vi "Orifice Flow Calculator of Water In Evaporation ASME.vi"(2 "Pipe Diameter (mm)":dbl[unit], 3 "Orifice Diameter":dbl[unit], 4 "Delta P\n(Presure Made By Orifice)":dbl[unit], 5 "Water Temperature":dbl[unit]=10.0 min=10.0 max=95.0) -> (0 "Iteration Volumetric Flow \n(Orifice) (Lit/min)":dbl[unit], 1 "Mass Flow (Orifice) (Kg/min)":dbl[unit])   [LabVIEW 2018]
panel:
  out "ReD":dbl
  out "Mass Flow (Orifice) (Kg/h)":dbl[unit](knob)
  out "Mass Flow (Orifice) (Kg/s)":dbl[unit]
  out "Pipe Velocity (m/s)":dbl[unit]
  out "Pipe Area (cm^2)":dbl[unit]
  out "Throat Velocity (m/s)":dbl[unit]
  out "Throat Area (cm^2)":dbl[unit]
  out "Beta":dbl
  out "orifice coefficient":dbl
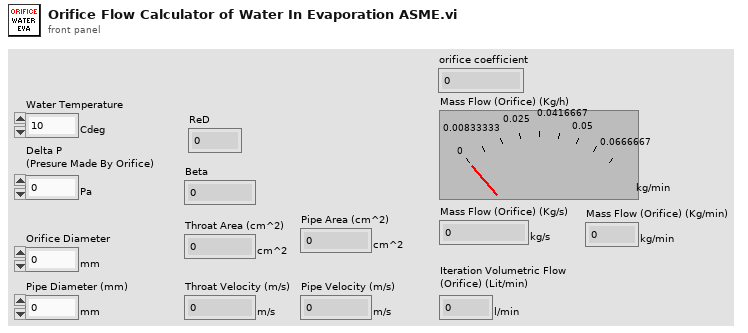
[diagram p1: front panel]
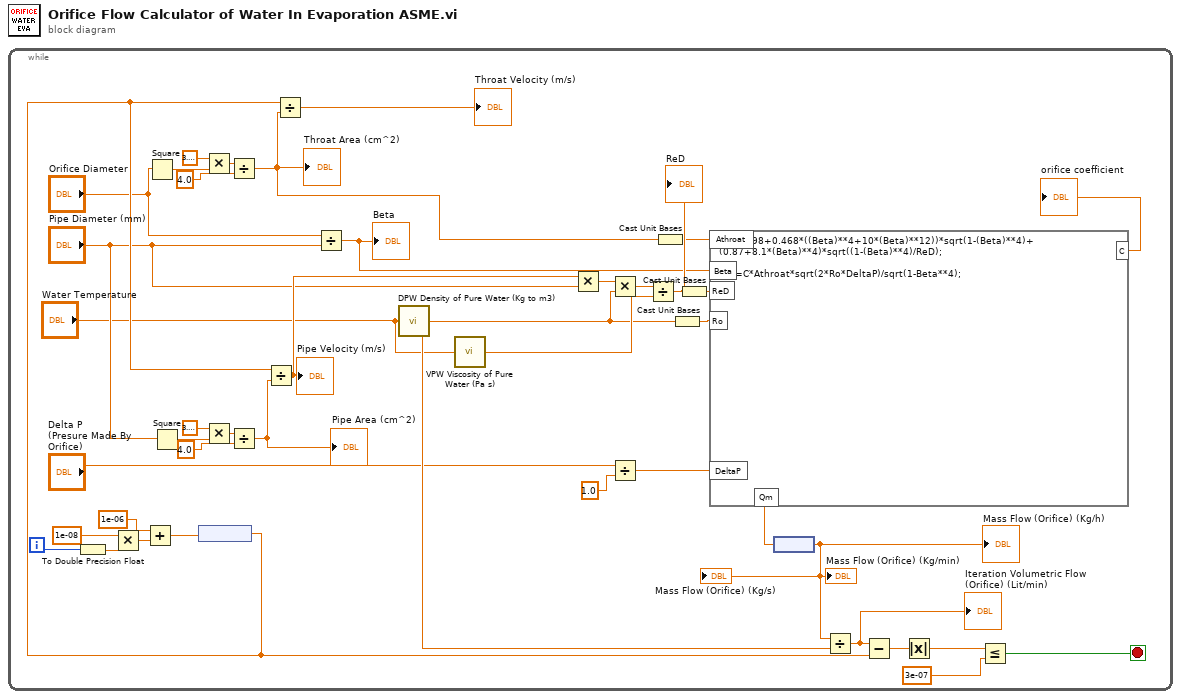
[diagram p0: block diagram]
diagram:
  n1 = while {
    i -> [w26]
    stop <- w19 stop-if-true
    n2 = To Double Precision Float(number=w26) -> (double precision float=w30:dbl)
    n3 = Multiply(x=1e-08, y=w30) -> (x*y=w28:dbl)
    n4 = Add(x=1e-06, y=w28) -> (x+y=w24:dbl)
    n5 = Square(x="Orifice Diameter") -> (x^2=w39:dbl[unit])
    n6 = Square(x="Pipe Diameter (mm)") -> (x^2=w35:dbl[unit])
    n7 = node(w24) -> (w23:dbl[unit])
    n8 = Multiply(x=3.141592653589793, y=w39) -> (x*y=w41:dbl[unit])
    n9 = Multiply(x=3.141592653589793, y=w35) -> (x*y=w37:dbl[unit])
    n10 = Divide(x=w41, y=4.0) -> (x/y=w11:dbl[unit])
    "Throat Area (cm^2)" <- w11
    n11 = Divide(x=w37, y=4.0) -> (x/y=w34:dbl[unit])
    "Pipe Area (cm^2)" <- w34
    n12 = Divide(x=w23, y=w34) -> (x/y=w7:dbl[unit])
    "Pipe Velocity (m/s)" <- w7
    n13 = Divide(x=w23, y=w11) -> (x/y=→"Throat Velocity (m/s)":dbl[unit])
    n14 = Divide(x="Orifice Diameter", y="Pipe Diameter (mm)") -> (x/y=w1:dbl)
    "Beta" <- w1
    n15 = call "DPW Density of Pure Water (Kg to m3).vi"("Pure Water Temprature"="Water Temperature") -> ("DPW"=w8:dbl[unit])
    n16 = call "VPW Viscosity of Pure Water (Pa s).vi"("Pure Water Temprature"="Water Temperature") -> ("Visocity of pure Water (Pa S)"=w13:dbl[unit])
    n17 = Multiply(x=w7, y="Pipe Diameter (mm)") -> (x*y=w18:dbl[unit])
    n18 = Multiply(x=w18, y=w8) -> (x*y=w17:dbl[unit])
    n19 = Divide(x="Delta P\n(Presure Made By Orifice)", y=dbl[unit] 1.0) -> (x/y=w2:dbl)
    n20 = Divide(x=w17, y=w13) -> (x/y=w15:dbl)
    "ReD" <- w15
    n21 = Cast Unit Bases(0:w11) -> (2:w12:dbl)  [unwired: 1 in]
    n22 = Cast Unit Bases(0:w8) -> (2:w9:dbl)  [unwired: 1 in]
    n23 = Cast Unit Bases(0:w15) -> (2:w14:dbl)  [unwired: 1 in]
    n24 = formula code="C=(0.598+0.468*((Beta)**4+10*(Beta)**12))*sqrt(1-(Beta)**4)+\n(0.87+8.1*(Beta)**4)*sqrt((1-(Beta)**4)/ReD);\n\nQm=C*Athroat*sqrt(2*Ro*DeltaP)/sqrt(1-Beta**4);"("Beta"=w1, "Athroat"=w12, "Ro"=w9, "DeltaP"=w2, "ReD"=w14) -> ("C"=→"orifice coefficient":dbl, "Qm"=w33:dbl)
    n25 = node(w33) -> (w31:dbl[unit])
    "Mass Flow (Orifice) (Kg/s)" <- w31
    "Mass Flow (Orifice) (Kg/h)" <- w31
    "Mass Flow (Orifice) (Kg/min)" <- w31
    n26 = Divide(x=w31, y=w8) -> (x/y=w25:dbl[unit])
    "Iteration Volumetric Flow \n(Orifice) (Lit/min)" <- w25
    n27 = Subtract(x=w25, y=w23) -> (x-y=w22:dbl[unit])
    n28 = Absolute Value(x=w22) -> (abs(x)=w21:dbl[unit])
    n29 = Less Or Equal?(x=w21, y=dbl[unit] 3e-07) -> (x <= y?=w19:bool)
  }
